vi "Type Conv - Dryer Cmd to String.vi"(11 "Dryer Cmd":T1=1 items=["CMD_Eval_Mode_Entry_CC1", "CMD_Eval_Mode_Entry_CC2", "CMD_Eval_Mode_Continue", "CMD_Send_DIAG_Info", "CMD_Enable_Debug_Log ", "CMD_Disable_Debug_Log ", "CMD_Send_Log_Data", "CMD_Stop", "RQST_Version"]) -> (3 "Read String":string)   [LabVIEW 2012]
uses:
  Dryer Commands.ctl
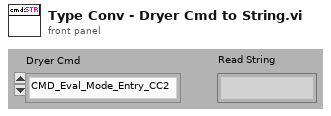
[diagram p1: front panel]
types:
  T1 = typedef "Dryer Commands.ctl" = u8
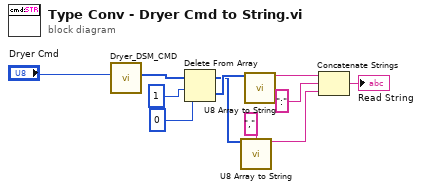
[diagram p0: block diagram]
diagram:
  n1 = call "Dryer_DSM_CMD.vi"("Command"="Dryer Cmd") -> ("CMD Array"=w2:u8[])  [unwired: 10 in]
  n2 = Delete From Array(array=w2, length=1, index=0) -> (deleted portion=w5:u8[], array with subset deleted=w4:u8[])
  n3 = call "U8 Array to String.vi"("U8 Data"=w4, "Delimiter(_)"=",") -> ("String"=w6:string)  [unwired: 13 in]
  n4 = call "U8 Array to String.vi"("U8 Data"=w5) -> ("String"=w8:string)  [unwired: 14 in]
  n5 = Concatenate Strings(w8, ":" ("string"), w6) -> (→"Read String":string)
